vi "Servo Read Pulse Width.vi"(0 "Arduino Resource":T1={"VISA resource"="", "Board Type"=enum."Arduino Uno", "Connection Type"=enum."USB / Serial", "Bytes Per Packet (15)"=15}, 5 "Servo Number":u8, 11 "error in":errorcluster) -> (4 "Arduino Resource":T1={"VISA resource"="", "Board Type"=enum."Arduino Uno", "Connection Type"=enum."USB / Serial", "Bytes Per Packet (15)"=15}, 8 "Pulse Width in uS":u16, 15 "error out":errorcluster)   [LabVIEW 2011, in "LabVIEW Interface for Arduino.lvlib"]
doc: "Reads the last pulse width, in uS, written to the specified servo."
uses:
  LabVIEW Interface for Arduino.lvlib
  Private/Type Defs/Arduino Resource.ctl
  Private/Type Defs/Board Type.ctl
  Private/Type Defs/Command.ctl
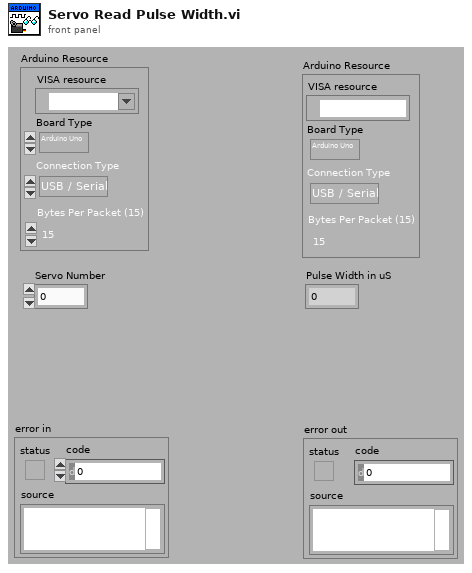
[diagram p1: front panel]
types:
  T1 = typedef "LabVIEW Interface for Arduino.lvlib/Arduino Resource.ctl" = cluster{"VISA resource":refnum<visa-resource-name>, "Board Type":T2, "Connection Type":enum8{"USB / Serial"}, "Bytes Per Packet (15)":u8}
  T2 = typedef "LabVIEW Interface for Arduino.lvlib/Board Type.ctl" = enum16{"Arduino Uno", "Dimuelanove w/Atmega 328", "Mega 2560", "Chipkit Uno32", "Chipkit Max32"}
  T3 = typedef "LabVIEW Interface for Arduino.lvlib/Command.ctl" = enum8{"setArduinoMode", "flushSerial", "setPinMode", "digitalWritePin", "digitalWritePort", "tone", "digitalReadPin", "digitalReadPort", "analogReadPin", "analogReadPort", "pwmWritePin", "pwmWritePort", "sevenSegment_Configure", "sevenSegment_Write", "I2C Init", "I2C Write", "I2C Read", "SPI Init", "SPI Set Bit Order", "SPI Set Clock Divider", "SPI Set Data Mode", "SPI Send / Receive", "SPI Close", "Servo Set Num Servos", "Servo Config Servo", "Servo Write Angle", "Servo Read Angle", "Servo Write Pulse Width", "Servo Read Pulse Width", "Servo Detach", "LCD Init", "LCD Set Size", "LCD Set Cursor Mode", "LCD Clear", "LCD Set Cursor Position", "LCD Print", "LCD Display Power", "LCD Scroll Display", "LCD Autoscroll", "LCD Print Direction", "LCD Create Custom Char", "LCD Print Custom Char", "contAcqOn", "contAcqOff", "getFirmwareVersion", "FiniteSampleStart"}
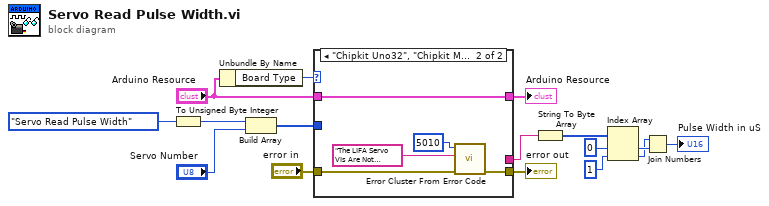
[diagram p0: block diagram]
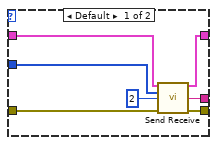
[diagram p2: hidden frame]
diagram:
  n1 = To Unsigned Byte Integer(number=Command."Servo Read Pulse Width" ("Command")) -> (unsigned 8bit integer=w15:u8)
  n2 = Unbundle By Name("Arduino Resource") -> ("Board Type"=w3:T2)
  n3 = Build Array(w15, "Servo Number") -> (w5:u8[])
  n4 = case shown="\"Chipkit Uno32\", \"Chipkit Max32\"" w3 {
    tunnel: "error in" -> [w22 w26]
    tunnel: [w20 w25] -> w4
    tunnel: "Arduino Resource" -> [w21 w24]
    tunnel: [w17 w24] -> w1
    tunnel: w5 -> [w19 _]
    tunnel: [w18 _] -> w7
    frame Default {
      n5 = call "Send Receive.vi"("Arduino Resource"=w21, "Data"=w19, "Bytes To Read (0)"=u8 2, "error in"=w22) -> ("Arduino Resource"=w17:T1, "Read Buffer"=w18:string, "error out"=w20:errorcluster)  [unwired: 9 in]
    }
    frame "Chipkit Uno32", "Chipkit Max32" {
      n6 = call <vilib>:"Error Cluster From Error Code.vi"("error in (no error)"=w26, "error message (\"\")"="The LIFA Servo VIs Are Not Supported On Chipkit Targets." ("source"), "error code (0)"=5010) -> ("error out"=w25:errorcluster)  [unwired: 6 in]
    }
  }
  "Arduino Resource" <- w1
  "error out" <- w4
  n7 = String To Byte Array(string=w7) -> (unsigned byte array=w13:u8[])
  n8 = Index Array(array=w13, index #1=0 ("index"), index #2=1 ("index")) -> (element #1=w10:u8, element #2=w9:u8)
  n9 = Join Numbers(hi=w9, lo=w10) -> ((hi.lo)=→"Pulse Width in uS":u16)
